vi "Find Owners.vi"(8 "error in (no error)":errorcluster, 11 "Array in":T1[](array[typedef])) -> (0 "error out":errorcluster, 3 "Array out":T1[](array[typedef]))   [LabVIEW 2023, in "VIDoc Parsing.lvlib" / "Structure Reporter.lvlib"]
uses:
  Structure Reporter.lvlib
  Structure Result 2.ctl
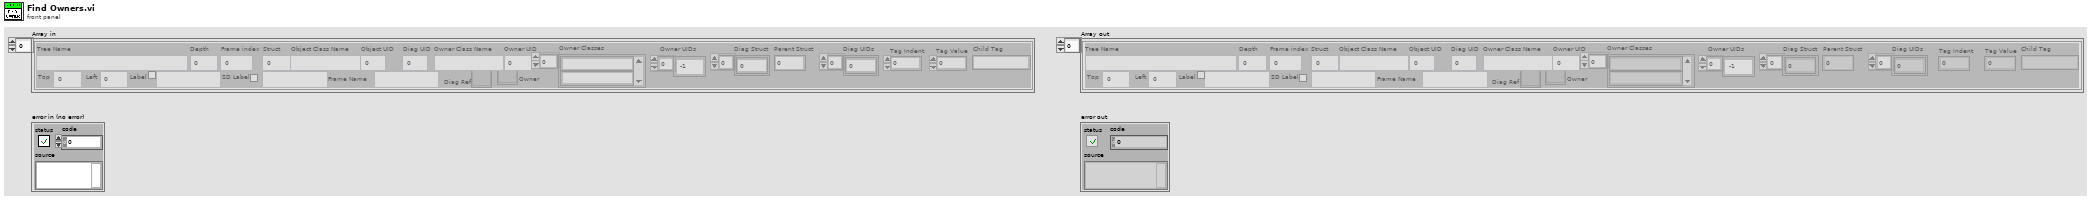
[diagram p1: front panel]
types:
  T1 = typedef "VIDoc Parsing.lvlib/Structure Reporter.lvlib/Structure Result 2.ctl" = cluster{"Depth":i32, "Top":i32, "Left":i32, "Frame index":i32, "Struct":i32, "Object Class Name":string, "Object UID":i32, "Label Visible":bool, "Object Label":string, "SD Label Visible":bool, "Object SD Label":string, "Frame Name":string, "Diag UID":i32, "Owner Class Name":string, "Owner UID":i32, "Diag Struct":i32[], "Parent Struct":i32, "Diag UIDs":i32[], "Tree Name":string, "Diag Ref":refnum<vi>, "Owner Classes":string[], "Owner":refnum<vi>, "Owner UIDs":i32[], "Tag Indent":i32, "Tag Value":i32, "Child Tag":string}
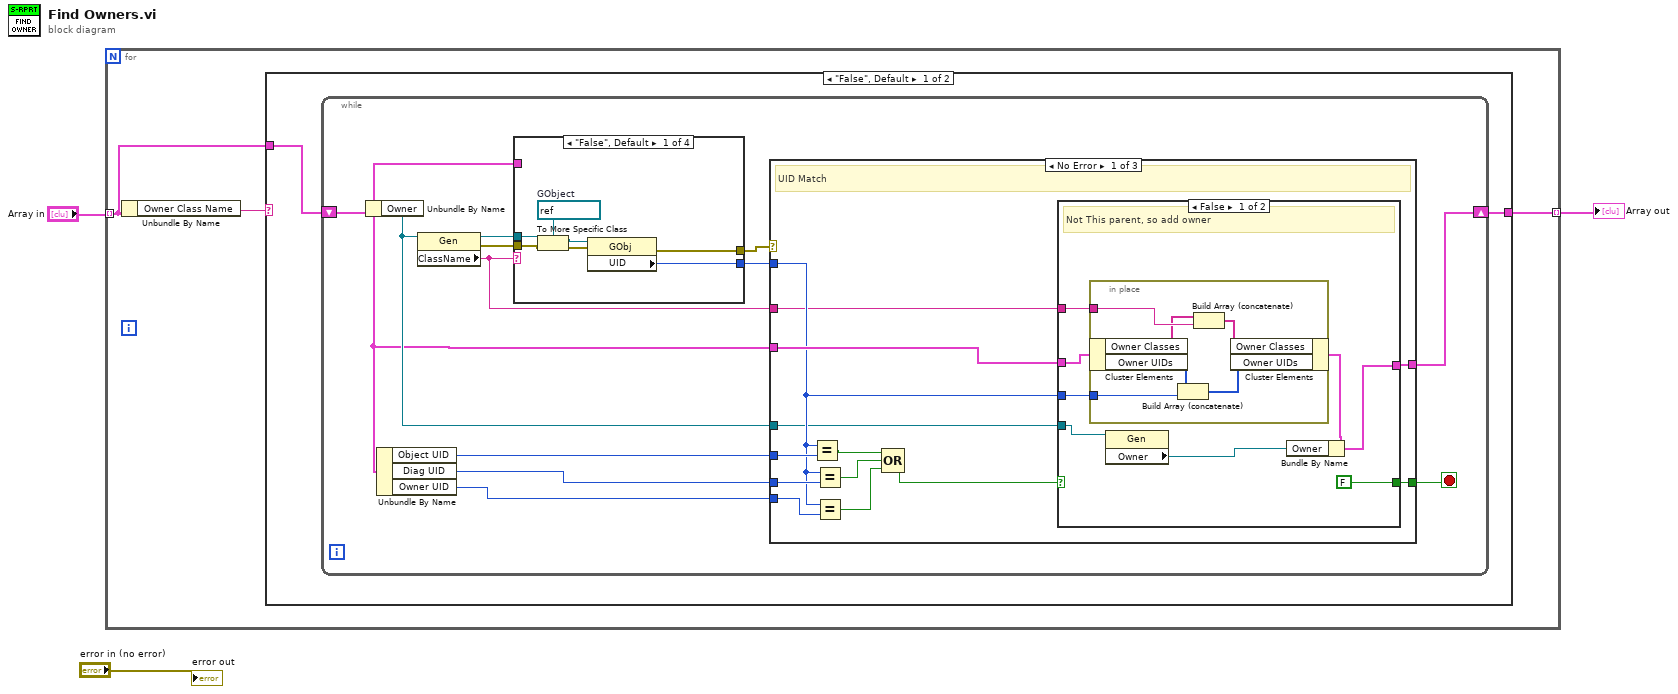
[diagram p0: block diagram]
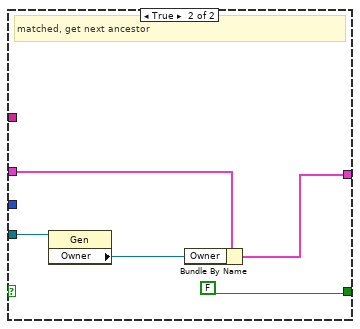
[diagram p2: hidden frame]
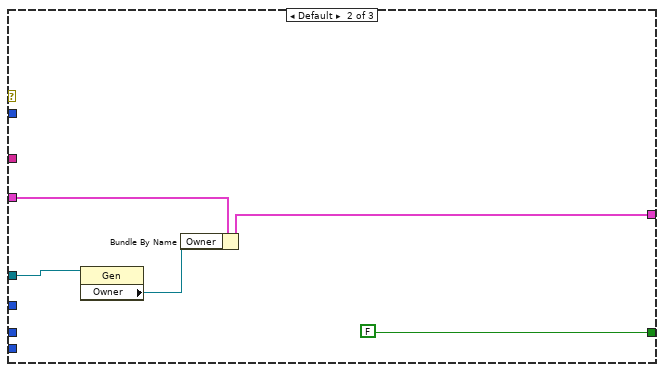
[diagram p3: hidden frame]
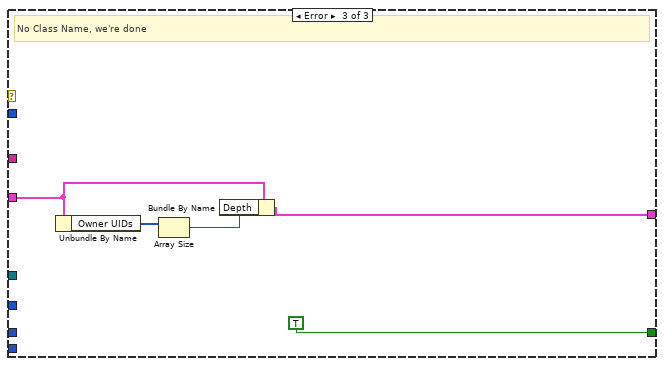
[diagram p4: hidden frame]
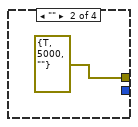
[diagram p5: hidden frame]
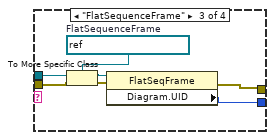
[diagram p6: hidden frame]
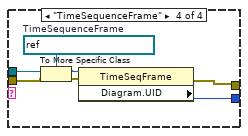
[diagram p7: hidden frame]
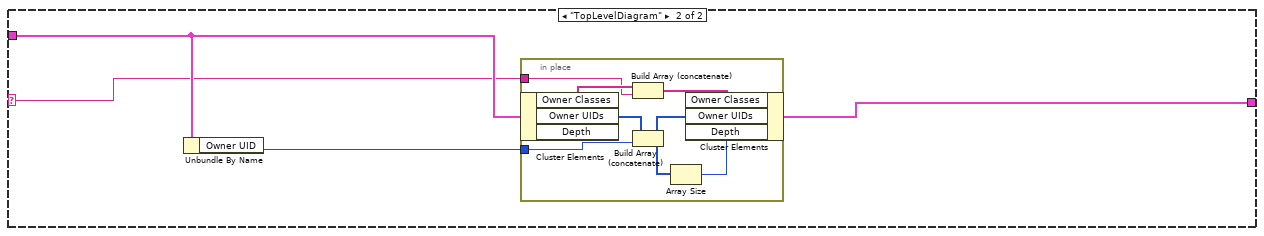
[diagram p8: hidden frame]
diagram:
  n1 = for {
    tunnel: "Array in" -> [w4] mode=indexing
    tunnel: [w5] -> w3 mode=indexing
    n2 = Unbundle By Name(w4) -> ("Owner Class Name"=w6:string)
    n3 = case shown="\"False\", Default" w6 {
      selector: w6 -> [_ w85]
      tunnel: w4 -> [w7 w87]
      tunnel: [w8 w86] -> w5
      frame "False", Default {
        n4 = while {
          shift-right: [w20] -> w8
          shift-left: w7 -> [w9]
          stop <- w15 stop-if-true
          n5 = Unbundle By Name(w9) -> ("Owner"=w14:refnum<vi>)
          n6 = Unbundle By Name(w9) -> ("Object UID"=w13:i32, "Diag UID"=w12:i32, "Owner UID"=w11:i32)
          n7 = property class="Gen"(reference=w14) -> (reference out=w19:refnum<vi>, error out=w18:errorcluster, "ClassName"=w10:string)  [unwired: 1 in]
          n8 = case shown="\"False\", Default" w10 {
            tunnel: w19 -> [w67 _ w75 w83]
            tunnel: w18 -> [w66 _ w74 w82]
            tunnel: [w64 _ w71 w79] -> w16
            tunnel: [w63 errorcluster {"status"=TRUE, "code"=5000, "source"=""} ("error out") w72 w80] -> w17
            tunnel: w9 -> [_ _ _ _]
            frame "False", Default {
              w69 = refnum<vi> refnum  # GObject
              n9 = To More Specific Class(target class=w69, reference=w67, error in=w66) -> (specific class reference=w68:refnum<vi>, error out=w65:errorcluster)
              n10 = property class="GObj"(reference=w68, error in=w65) -> (error out=w63:errorcluster, "UID"=w64:i32)  [unwired: 1 out]
            }
            frame "" {
            }
            frame "FlatSequenceFrame" {
              w76 = refnum<vi> refnum  # FlatSequenceFrame
              n11 = To More Specific Class(target class=w76, reference=w75, error in=w74) -> (specific class reference=w77:refnum<vi>, error out=w73:errorcluster)
              n12 = property class="FlatSeqFrame"(reference=w77, error in=w73) -> (error out=w72:errorcluster, "Diagram.UID"=w71:i32)  [unwired: 1 out]
            }
            frame "TimeSequenceFrame" {
              w78 = refnum<vi> refnum  # TimeSequenceFrame
              n13 = To More Specific Class(target class=w78, reference=w83, error in=w82) -> (specific class reference=w84:refnum<vi>, error out=w81:errorcluster)
              n14 = property class="TimeSeqFrame"(reference=w84, error in=w81) -> (error out=w80:errorcluster, "Diagram.UID"=w79:i32)  [unwired: 1 out]
            }
          }
          n15 = case shown="No Error" w17 {
            tunnel: [w33 w53 w58] -> w20
            tunnel: w16 -> [w23 _ _]
            tunnel: w9 -> [w31 w54 w60]
            tunnel: [w32 FALSE TRUE] -> w15
            tunnel: w14 -> [w22 w55 _]
            tunnel: w13 -> [w30 _ _]
            tunnel: w12 -> [w29 _ _]
            tunnel: w11 -> [w28 _ _]
            tunnel: w10 -> [w21 _ _]
            frame No Error {
              # "UID Match"
              n16 = Equal?(x=w23, y=w30) -> (x = y?=w27:bool)
              n17 = Equal?(x=w23, y=w29) -> (x = y?=w26:bool)
              n18 = Equal?(x=w23, y=w28) -> (x = y?=w25:bool)
              n19 = Compound Arithmetic op=OR(w27, w26, w25) -> (w24:bool)
              n20 = case shown="False" w24 {
                tunnel: w31 -> [w41 w49]
                tunnel: [w35 w51] -> w33
                tunnel: [FALSE FALSE] -> w32
                tunnel: w23 -> [w40 _]
                tunnel: w22 -> [w37 w50]
                tunnel: w21 -> [w34 _]
                frame False {
                  # "Not This parent, so add owner"
                  n21 = in-place {
                    in-place-border: w40 -> [w45]
                    in-place-border: w34 -> [w44]
                    n22 = in-place-cluster #1(w41) -> ("Owner Classes"=w43:string[], "Owner UIDs"=w47:i32[])
                    n23 = Build Array (concatenate)(w47, w45) -> (w46:i32[])
                    n24 = Build Array (concatenate)(w43, w44) -> (w42:string[])
                    n25 = in-place-cluster #1("Owner Classes"=w42, "Owner UIDs"=w46) -> (w36:T1)
                  }
                  n26 = property class="Gen"(reference=w37) -> ("Owner"=w38:refnum<vi>)  [unwired: 1 in, 2 out]
                  n27 = Bundle By Name(cluster=w36, "Owner"=w38) -> (w35:T1)
                }
                frame True {
                  # "matched, get next ancestor"
                  n28 = property class="Gen"(reference=w50) -> ("Owner"=w52:refnum<vi>)  [unwired: 1 in, 2 out]
                  n29 = Bundle By Name(cluster=w49, "Owner"=w52) -> (w51:T1)
                }
              }
            }
            frame Default {
              n30 = property class="Gen"(reference=w55) -> ("Owner"=w56:refnum<vi>)  [unwired: 1 in, 2 out]
              n31 = Bundle By Name(cluster=w54, "Owner"=w56) -> (w53:T1)
            }
            frame Error {
              # "No Class Name, we're done"
              n32 = Unbundle By Name(w60) -> ("Owner UIDs"=w61:i32[])
              n33 = Array Size(array=w61) -> (size(s)=w59:i32)
              n34 = Bundle By Name(cluster=w60, "Depth"=w59) -> (w58:T1)
            }
          }
        }
      }
      frame "TopLevelDiagram" {
        n35 = Unbundle By Name(w87) -> ("Owner UID"=w88:i32)
        n36 = in-place {
          in-place-border: w88 -> [w94]
          in-place-border: w85 -> [w91]
          n37 = in-place-cluster #2(w87) -> ("Owner Classes"=w93:string[], "Owner UIDs"=w95:i32[])  [unwired: 1 out]
          n38 = Build Array (concatenate)(w93, w91) -> (w92:string[])
          n39 = Build Array (concatenate)(w95, w94) -> (w90:i32[])
          n40 = Array Size(array=w90) -> (size(s)=w89:i32)
          n41 = in-place-cluster #2("Owner Classes"=w92, "Owner UIDs"=w90, "Depth"=w89) -> (w86:T1)
        }
      }
    }
  }
  "Array out" <- w3
  "error out" <- "error in (no error)"
